vi "CONV 2D Fractional Array to String.vi"(0 "2-D Fractional":dbl[][](array[numeric]) format="%.2f", 1 "Delimiters (,;)":string=",;", 5 "Precision (2)":i16=2) -> (6 "String":string)   [LabVIEW 2012]
doc: "This routine converts a 2-D DBL Precision Fractional Array into a String list. There must be exactly 2 characters in the delimiters field. The first character is the Column Delimiter, and the second character is the Row Delimiter.\n\nExample:\n\n2-D String Input:\n\n1 2 3\n4 5 6\n\nDelimiters:\n,;\n\nString Output:\n\n1,2,3;4,5,6"
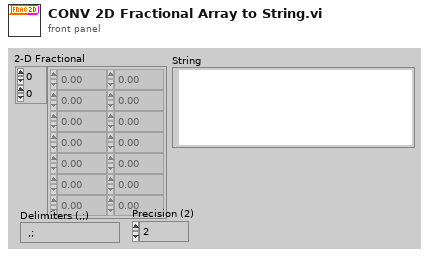
[diagram p1: front panel]
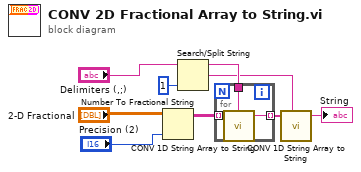
[diagram p0: block diagram]
diagram:
  n1 = Number To Fractional String(number="2-D Fractional", precision (6)="Precision (2)") -> (F-format string=w3:string[][])  [unwired: 2 out]
  n2 = Search/Split String(string="Delimiters (,;)", offset (0)=1) -> (substring before match=w5:string, match + rest of string=w4:string)  [unwired: 2 out]
  n3 = for {
    tunnel: w3 -> [w12] mode=indexing
    tunnel: [w11] -> w9 mode=indexing
    tunnel: w5 -> [w10]
    n4 = call "CONV 1D String Array to String.vi"("1-D String"=w12, "Delimiter (,)"=w10) -> ("String"=w11:string)  [unwired: 7 out]
  }
  n5 = call "CONV 1D String Array to String.vi"("1-D String"=w9, "Delimiter (,)"=w4) -> ("String"=→"String":string)  [unwired: 7 out]
